vi "Get Thread Reference.vi"(8 "error in (no error)":errorcluster, 11 "Thing in":refnum<class "Server.lvclass">) -> (0 "error out":errorcluster, 1 "Thread VI":refnum<vi>, 3 "Thing out":refnum<class "Server.lvclass">)   [LabVIEW 2023]
uses:
  Server.lvclass
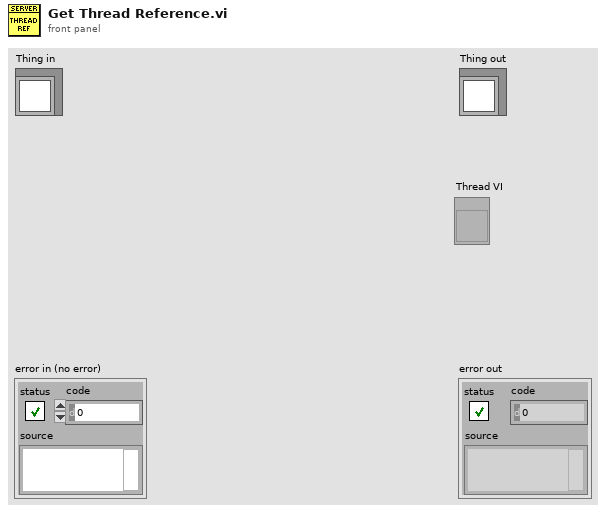
[diagram p1: front panel]
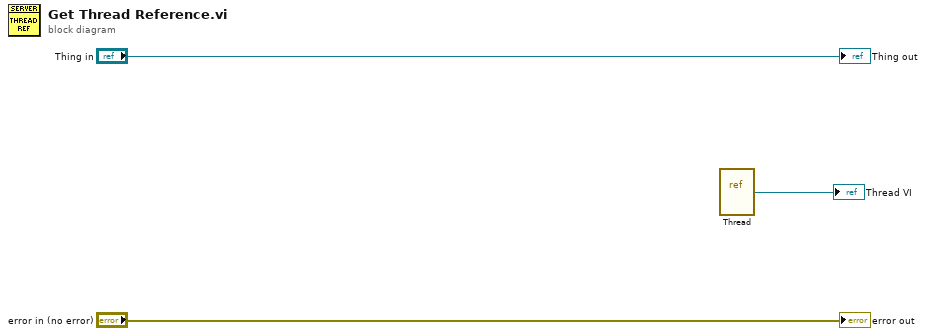
[diagram p0: block diagram]
diagram:
  n1 = vi-ref "Thread.vi"() -> (→"Thread VI":refnum<vi>)
  "error out" <- "error in (no error)"
  "Thing out" <- "Thing in"
